vi "Write Value.vi"(8 "error in (no error)":errorcluster, 10 "Value":dbl, 11 "DBL Result in":refnum<class "DBL Payload.lvclass">) -> (0 "error out":errorcluster, 3 "DBL Result out":refnum<class "DBL Payload.lvclass">)   [LabVIEW 2015, in "DBL Payload.lvclass"]
uses:
  DBL Payload.lvclass
  DBL Payload.lvclass/DBL Payload.ctl
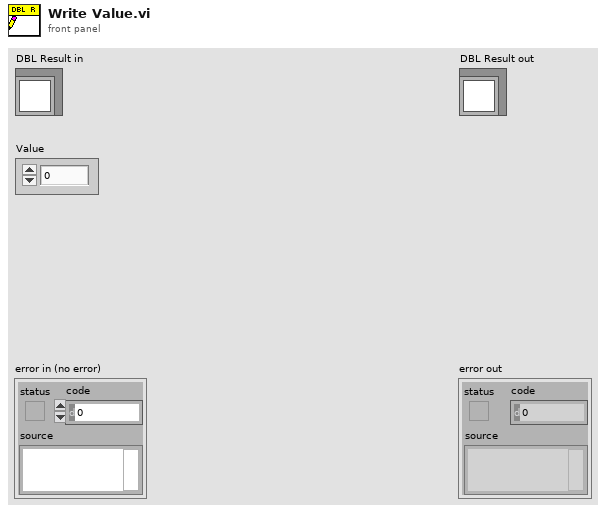
[diagram p1: front panel]
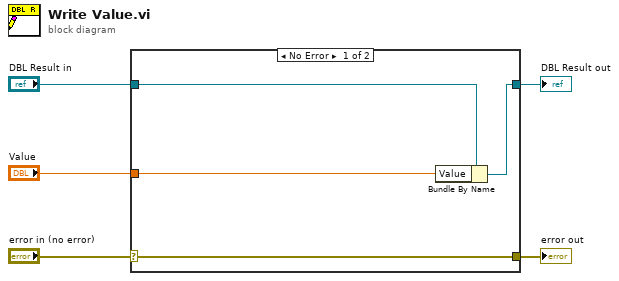
[diagram p0: block diagram]
diagram:
  n1 = case shown="No Error" "error in (no error)" {
    selector: "error in (no error)" -> [w9 w10]
    tunnel: [w9 w10] -> w4
    tunnel: [w7 w11] -> w2
    tunnel: "DBL Result in" -> [w8 w11]
    tunnel: "Value" -> [w6 _]
    frame No Error {
      n2 = Bundle By Name(cluster=w8, "Value"=w6) -> (w7:refnum<class "DBL Payload.lvclass">)
    }
    frame Error {
    }
  }
  "error out" <- w4
  "DBL Result out" <- w2
